vi "Start CLI Interface.vi"(8 "error in (no error)":errorcluster) -> (0 "error out":errorcluster, 1 "Working Directory":path, 2 "Custom Parameters":string[](array[string]), 3 "CLI out":refnum<class "CLI.lvclass">, 5 "Events Regs.":refnum<event-registration>)   [LabVIEW 2024, in "CLI.lvclass"]
doc: "Starts the connection to the command line.\n\n<b>Custom Parameters</b> will return the command line parameters passed for your application."
uses:
  CLI.lvclass
  CLI.lvclass/CLI.ctl
  Signal Loop.vi
  Events.ctl
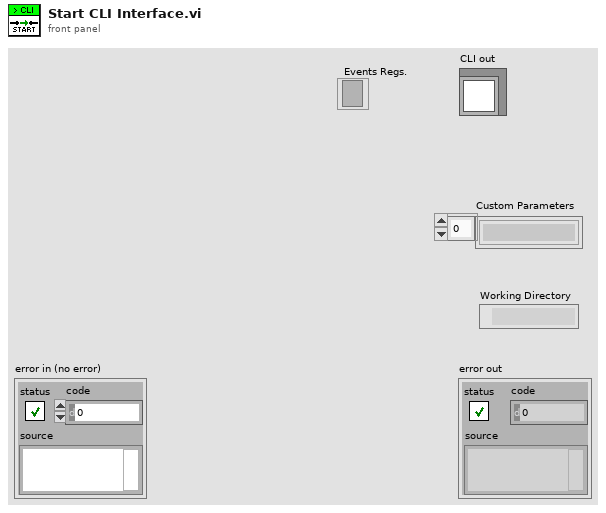
[diagram p1: front panel]
types:
  T1 = typedef "Events.ctl" = cluster{"STIN":refnum<user-event>, "SIGI":refnum<user-event>, "UnknownSignal":refnum<user-event>}
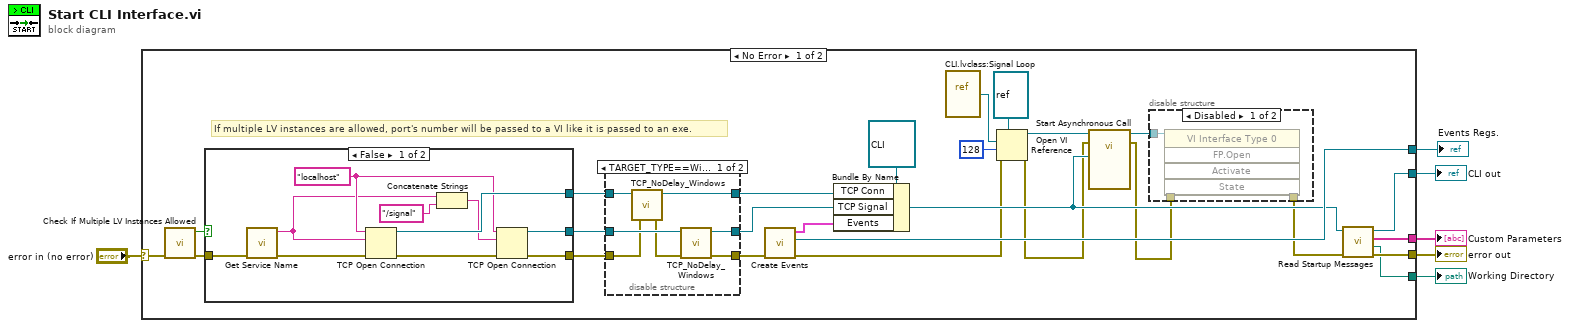
[diagram p0: block diagram]
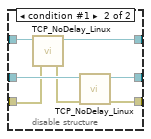
[diagram p3: hidden frame]
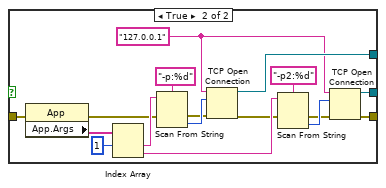
[diagram p4: hidden frame]
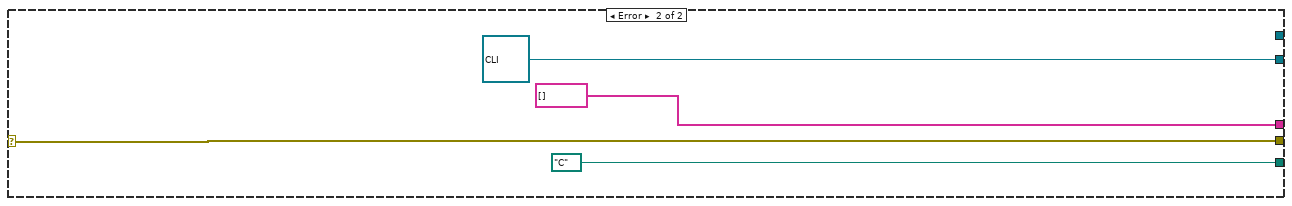
[diagram p5: hidden frame]
diagram:
  n1 = case shown="No Error" "error in (no error)" {
    selector: "error in (no error)" -> [w32 w81]
    tunnel: [w30 w81] -> w2
    tunnel: [w29 refnum<class "CLI.lvclass"> refnum ("CLI in")] -> w3
    tunnel: [w28 string[] []] -> w5
    tunnel: [w27 path "C:/" ("Working Directory")] -> w4
    tunnel: [w18 _] -> w1
    frame No Error {
      # "If multiple LV instances are allowed, port's number will be passed to a VI like it is passed to an exe."
      n2 = call "Check If Multiple LV Instances Allowed.vi"("error in"=w32) -> ("error out"=w24:errorcluster, "Multiple LV Instances allowed?"=w14:bool)  [unwired: 9 in]
      n3 = case shown="False" w14 {
        tunnel: w24 -> [w59 w70]
        tunnel: [w55 w61] -> w23
        tunnel: [w58 w69] -> w22
        tunnel: [w51 w68] -> w21
        frame False {
          w56 = "localhost" ("address")
          n4 = call "Get Service Name.vi"("error in (no error)"=w59) -> ("error out"=w60:errorcluster, "Service Name"=w54:string)  [unwired: 9 in]
          n5 = TCP Open Connection(address=w56, remote port or service name=w54, error in (no error)=w60) -> (connection ID=w58:refnum<k5>, error out=w57:errorcluster)  [unwired: 2 in]
          n6 = Concatenate Strings(w54, "/signal" ("string")) -> (w53:string)
          n7 = TCP Open Connection(address=w56, remote port or service name=w53, error in (no error)=w57) -> (connection ID=w51:refnum<k5>, error out=w55:errorcluster)  [unwired: 2 in]
        }
        frame True {
          w67 = "127.0.0.1" ("address")
          n8 = property class="App"(error in=w70) -> (error out=w71:errorcluster, "App.Args"=w72:string[])  [unwired: 1 in, 1 out]
          n9 = Index Array(array=w72, index #1=1 ("index")) -> (element #1=w75:string, element #2=w65:string)  [unwired: 1 in]
          n10 = Scan From String(format string="-p:%d", input string=w75, error in=w71) -> (error out=w73:errorcluster, output 1=w74:i32)  [unwired: 2 in, 2 out]
          n11 = TCP Open Connection(address=w67, remote port or service name=w74, error in (no error)=w73) -> (connection ID=w69:refnum<k5>, error out=w63:errorcluster)  [unwired: 2 in]
          n12 = Scan From String(format string="-p2:%d", input string=w65, error in=w63) -> (error out=w62:errorcluster, output 1=w64:i32)  [unwired: 2 in, 2 out]
          n13 = TCP Open Connection(address=w67, remote port or service name=w64, error in (no error)=w62) -> (connection ID=w68:refnum<k5>, error out=w61:errorcluster)  [unwired: 2 in]
        }
      }
      n14 = disable-structure shown="TARGET_TYPE==Windows, Default" {
        disable-tunnel: [w43 w49] -> w26
        disable-tunnel: [w37 w46] -> w25
        disable-tunnel: w23 -> [w39 w45]
        disable-tunnel: w22 -> [w42 w50]
        disable-tunnel: w21 -> [w41 w48]
        disable-tunnel: [w40 w47] -> w20
        frame condition #0 (active) {
          n15 = call "TCP_NoDelay_Windows.vi"("error in (no error)"=w39, "connID"=w42) -> ("error out"=w38:errorcluster, "connID 2"=w43:refnum<k5>)  [unwired: 4 in]
          n16 = call "TCP_NoDelay_Windows.vi"("error in (no error)"=w38, "connID"=w41) -> ("error out"=w37:errorcluster, "connID 2"=w40:refnum<k5>)  [unwired: 4 in]
        }
        frame condition #1 {
          n17 = call "TCP_NoDelay_Linux.vi"("error in (no error)"=w45, "connID"=w50) -> ("error out"=w44:errorcluster, "connID 2"=w49:refnum<k5>)  [unwired: 4 in]
          n18 = call "TCP_NoDelay_Linux.vi"("error in (no error)"=w44, "connID"=w48) -> ("error out"=w46:errorcluster, "connID 2"=w47:refnum<k5>)  [unwired: 4 in]
        }
      }
      n19 = call "Create Events.vi"("error in (no error)"=w25) -> ("error out"=w16:errorcluster, "Event Regs"=w18:refnum<event-registration>, "Events"=w19:T1)  [unwired: 8 in]
      n20 = Bundle By Name(cluster=refnum<class "CLI.lvclass"> refnum ("CLI in"), "TCP Conn"=w26, "TCP Signal"=w20, "Events"=w19) -> (w17:refnum<class "CLI.lvclass">)
      n21 = vi-ref "CLI.lvclass:Signal Loop.vi"() -> (w12:refnum<vi>)
      n22 = Open VI Reference(type specifier VI Refnum (for type only)=refnum<vi> refnum, vi path=w12, options=128, error in (no error)=w16) -> (vi reference=w10:refnum<vi>, error out=w9:errorcluster)  [unwired: 2 in]
      n23 = call-by-ref "Start Asynchronous Call"(reference=w10, error in=w9, "CLI in"=w17) -> (reference out=w7:refnum<vi>, error out=w8:errorcluster)  [unwired: 10 in, 1 out]
      n24 = disable-structure shown="Disabled" {
        disable-tunnel: [w35 w36] -> w15
        disable-tunnel: w8 -> [w34 w36]
        disable-tunnel: w7 -> [w33 _]
        frame Disabled {
          n25 = invoke class="VI Interface Type 0" method="FP.Open"(reference=w33, error in=w34) -> (error out=w35:errorcluster)  [unwired: 3 in, 4 out]
        }
        frame Enabled {
        }
      }
      n26 = call "Read Startup Messages.vi"("error in (no error)"=w15, "CLI in"=w17) -> ("error out"=w30:errorcluster, "Working Directory"=w27:path, "Arguments"=w28:string[], "CLI out"=w29:refnum<class "CLI.lvclass">)  [unwired: 6 in]
    }
    frame Error {
    }
  }
  "error out" <- w2
  "CLI out" <- w3
  "Custom Parameters" <- w5
  "Working Directory" <- w4
  "Events Regs." <- w1
